vi "rsp_Incompatible DC Connection.vi"(4 "Show in Debugger?":bool=TRUE, 6 "Message Priority":T1=enum."Normal", 8 "error in":errorcluster, 9 "Data in":T2, 11 "DS TCP Server in":refnum<class "DS TCP Server.lvclass">) -> (0 "error out":errorcluster, 3 "dup DS TCP Server out":refnum<class "DS TCP Server.lvclass">)   [LabVIEW 2017, in "DS TCP Server.lvlib" / "DS TCP Server.lvclass"]
doc: "This VI sends a <b>Public API Response</b> message to a registered MHL case of the Caller of the Worker that owns this VI.\n---"
uses:
  DS TCP Server.lvclass
  C:/Program Files (x86)/National Instruments/LabVIEW 2017/vi.lib/addons/_Workers/Library/Classes/Worker/Worker.lvclass
  rsp_Incompatible DC Connection.ctl
  <vilib>/addons/_Workers/Library/Classes/Message/Priority.ctl
  DS TCP Server.lvclass/DS TCP Server.ctl
  <vilib>/Utility/error.llb/Error Cluster From Error Code.vi
  <vilib>/ErrorRing/Error Ring.xnode
  <vilib>/addons/_Workers/Library/Classes/Message Queue/Message Queue.lvclass
  <vilib>/addons/_Workers/Library/Classes/Worker/Worker.lvclass
  <vilib>/addons/_Workers/Library/Classes/Message/Message.lvclass
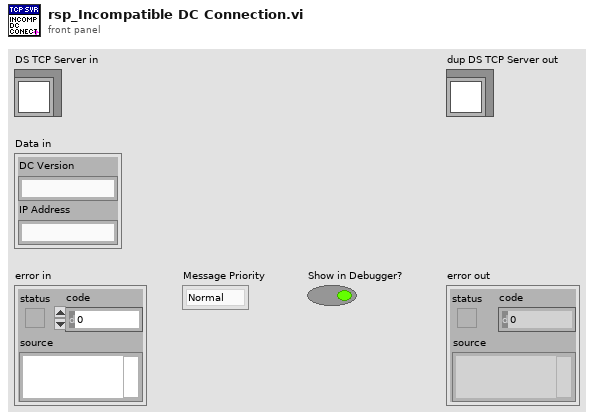
[diagram p1: front panel]
types:
  T1 = typedef "Workers.lvlib/Message.lvclass/Priority.ctl" = enum16{"Low", "Normal", "High"}
  T2 = typedef "DS TCP Server.lvlib/DS TCP Server.lvclass/rsp_Incompatible DC Connection.ctl" = cluster{"DC Version":string, "IP Address":string}
  T3 = typedef "Workers.lvlib/Case Label.ctl" = string
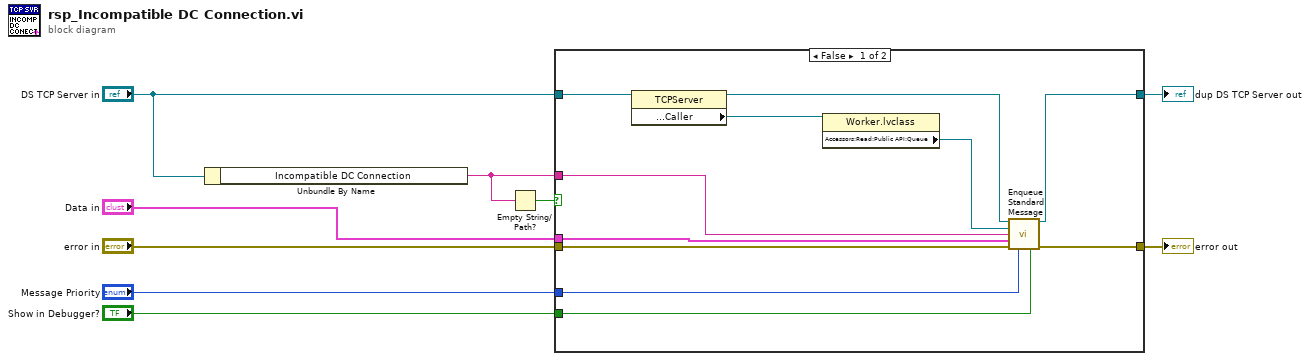
[diagram p0: block diagram]
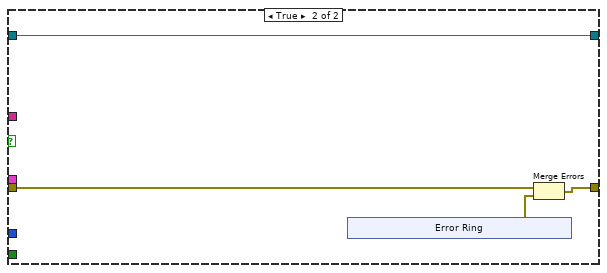
[diagram p2: hidden frame]
diagram:
  n1 = Unbundle By Name("DS TCP Server in") -> ("Incompatible DC Connection"=w4:T3)
  n2 = Empty String/Path?(string/path=w4) -> (empty?=w5:bool)
  n3 = case shown="False" w5 {
    tunnel: "error in" -> [w19 w21]
    tunnel: [w18 w22] -> w8
    tunnel: "Data in" -> [w15 _]
    tunnel: [w17 w24] -> w6
    tunnel: "DS TCP Server in" -> [w20 w24]
    tunnel: w4 -> [w16 _]
    tunnel: "Show in Debugger?" -> [w14 _]
    tunnel: "Message Priority" -> [w13 _]
    frame False {
      n4 = property class="TCPServer"(reference=w20) -> (reference out=w12:refnum<class "DS TCP Server.lvclass">, "Accessors:Read:Public API:Caller"=w11:refnum<class "Worker.lvclass">)  [unwired: 1 in, 1 out]
      n5 = property class="Worker.lvclass"(reference=w11) -> ("Accessors:Read:Public API:Queue"=w10:refnum<class "Message Queue.lvclass">)  [unwired: 1 in, 2 out]
      n6 = call-dynamic "Enqueue Standard Message.vi"("Worker"=w12, "Message Queue"=w10, "Case Label"=w16, "Data"=w15, "error in (no error)"=w19, "Priority (Normal)"=w13, "Send Message to Debugger? (T)"=w14) -> ("dup Worker out"=w17:refnum<class "DS TCP Server.lvclass">, "error out"=w18:errorcluster)  [unwired: 7 in]
    }
    frame True {
      n7 = xnode "Error Ring"() -> ("error out"=w23:errorcluster)
      n8 = Merge Errors(w21, w23) -> (w22:errorcluster)
    }
  }
  "error out" <- w8
  "dup DS TCP Server out" <- w6
